vi "Columns.vi"() -> (2 "Columns":T1)   [LabVIEW 2020, in "tests.lvlib" / "Test2.lvclass"]
uses:
  Test2.lvclass
  Columns.ctl
  <vilib>/IlluminatedG/IG Conditum Base/Conditum/Columns/Integer/Integer.lvclass
  Test2.lvclass/Test2.ctl
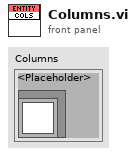
[diagram p1: front panel]
types:
  T1 = typedef "tests.lvlib/Test2.lvclass/Columns.ctl" = cluster{"<Placeholder>":refnum<class "Integer.lvclass">}
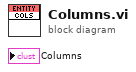
[diagram p0: block diagram]
diagram:
